vi "RichToFlatgrpc_reflection_v1alpha_ServiceResponse.vi"(5 "OutputClusterType":T1, 11 "InputCluster":T2) -> (3 "OutputCluster":T1)   [LabVIEW 2025, in "reflection_server.lvlib"]
uses:
  reflection_server.lvlib
  grpc_reflection_v1alpha_ServiceResponse.ctl
  grpc_reflection_v1alpha_ServiceResponse_Flat.ctl
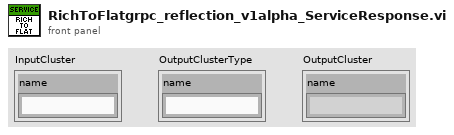
[diagram p1: front panel]
types:
  T1 = typedef "reflection_server.lvlib/grpc_reflection_v1alpha_ServiceResponse_Flat.ctl" = cluster{"name":string}
  T2 = typedef "reflection_server.lvlib/grpc_reflection_v1alpha_ServiceResponse.ctl" = cluster{"name":string}
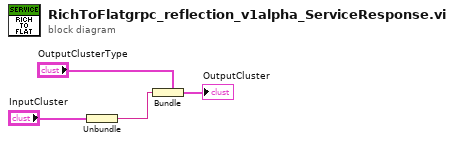
[diagram p0: block diagram]
diagram:
  n1 = Unbundle "Unbundle"("InputCluster") -> ("name"=w1:string)
  n2 = Bundle "Bundle"(cluster="OutputClusterType", "name"=w1) -> (→"OutputCluster":T1)
